vi "Get Class Name.vi"(8 "error in (no error)":errorcluster, 11 "object":refnum<class>) -> (0 "error out":errorcluster, 3 "Class Name":string)   [LabVIEW 2026, in "TALOS.lvlib"]
doc: "This VI returns the name of the class given in input (without the .lvclass extension)."
uses:
  TALOS.lvlib
  <vilib>/AdvancedString/Delimited String to 1D String Array (string).vi
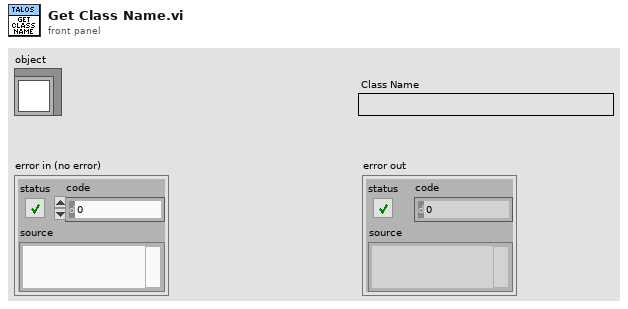
[diagram p1: front panel]
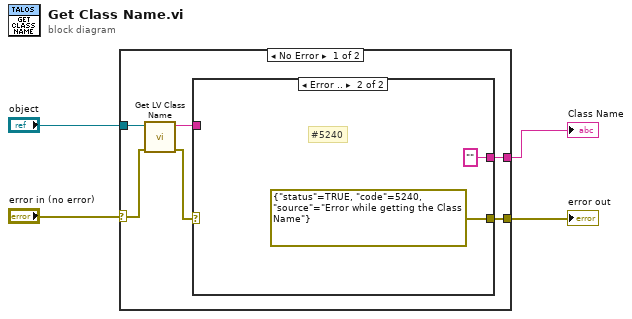
[diagram p0: block diagram]
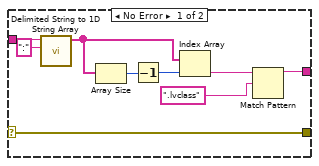
[diagram p2: hidden frame]
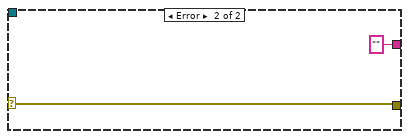
[diagram p3: hidden frame]
diagram:
  n1 = case shown="No Error" "error in (no error)" {
    selector: "error in (no error)" -> [w7 w22]
    tunnel: [w9 "" ("String")] -> w4
    tunnel: "object" -> [w8 _]
    tunnel: [w6 w22] -> w1
    frame No Error {
      n2 = call <vilib>:"Get LV Class Name.vi"("error in (no error)"=w7, "object"=w8) -> ("error out"=w5:errorcluster, "class name"=w10:string)  [unwired: 8 in]
      n3 = case shown="Error .." w5 {
        selector: w5 -> [w11 _]
        tunnel: w10 -> [w19 _]
        tunnel: [w14 "" ("String")] -> w9
        tunnel: [w11 errorcluster {"status"=TRUE, "code"=5240, "source"="Error while getting the Class Name"} ("error IO")] -> w6
        frame No Error {
          n4 = call-poly <vilib>:"Delimited String to 1D String Array.vi"("delimiter"=":", "delimited string"=w19) -> ("string array"=w16:string[])  [unwired: 9 in]
          n5 = Array Size(array=w16) -> (size(s)=w17:i32)
          n6 = Decrement(x=w17) -> (x-1=w15:i32)
          n7 = Index Array(array=w16, index=w15) -> (element=w13:string)
          n8 = Match Pattern(string=w13, regular expression=".lvclass") -> (before substring=w14:string)  [unwired: 1 in, 3 out]
        }
        frame Error {
          # "#5240"
        }
      }
    }
    frame Error {
    }
  }
  "Class Name" <- w4
  "error out" <- w1
